vi "Cooling monitor.vi"() -> ()   [LabVIEW 2024]
panel:
  out "Humidity":dbl
  out "Fan steps":dbl
  out "Max Temp":dbl
  out "Min Temp":dbl
  out "Get Arduino Data":bool
  out "Fan Status":bool
  out "Waveform Chart":cluster{"x+y":dbl, dbl, dbl}(graph)
  out "Humidity":dbl(slide) scale=0.0..100.0 scale format="%.0p"
  out "Thermometer":dbl(slide) scale=0.0..100.0
  out "Fan status":string
  out "Humidity":string
  out "Temp":string
  out "Date and time":string
  in  "stop":bool
  out "error out":errorcluster
  out "read buffer":string
  in  "VISA resource name":refnum<visa-resource-name>="COM7"
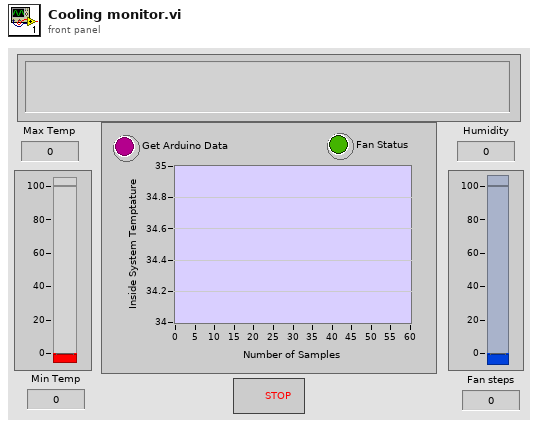
[diagram p1: front panel]
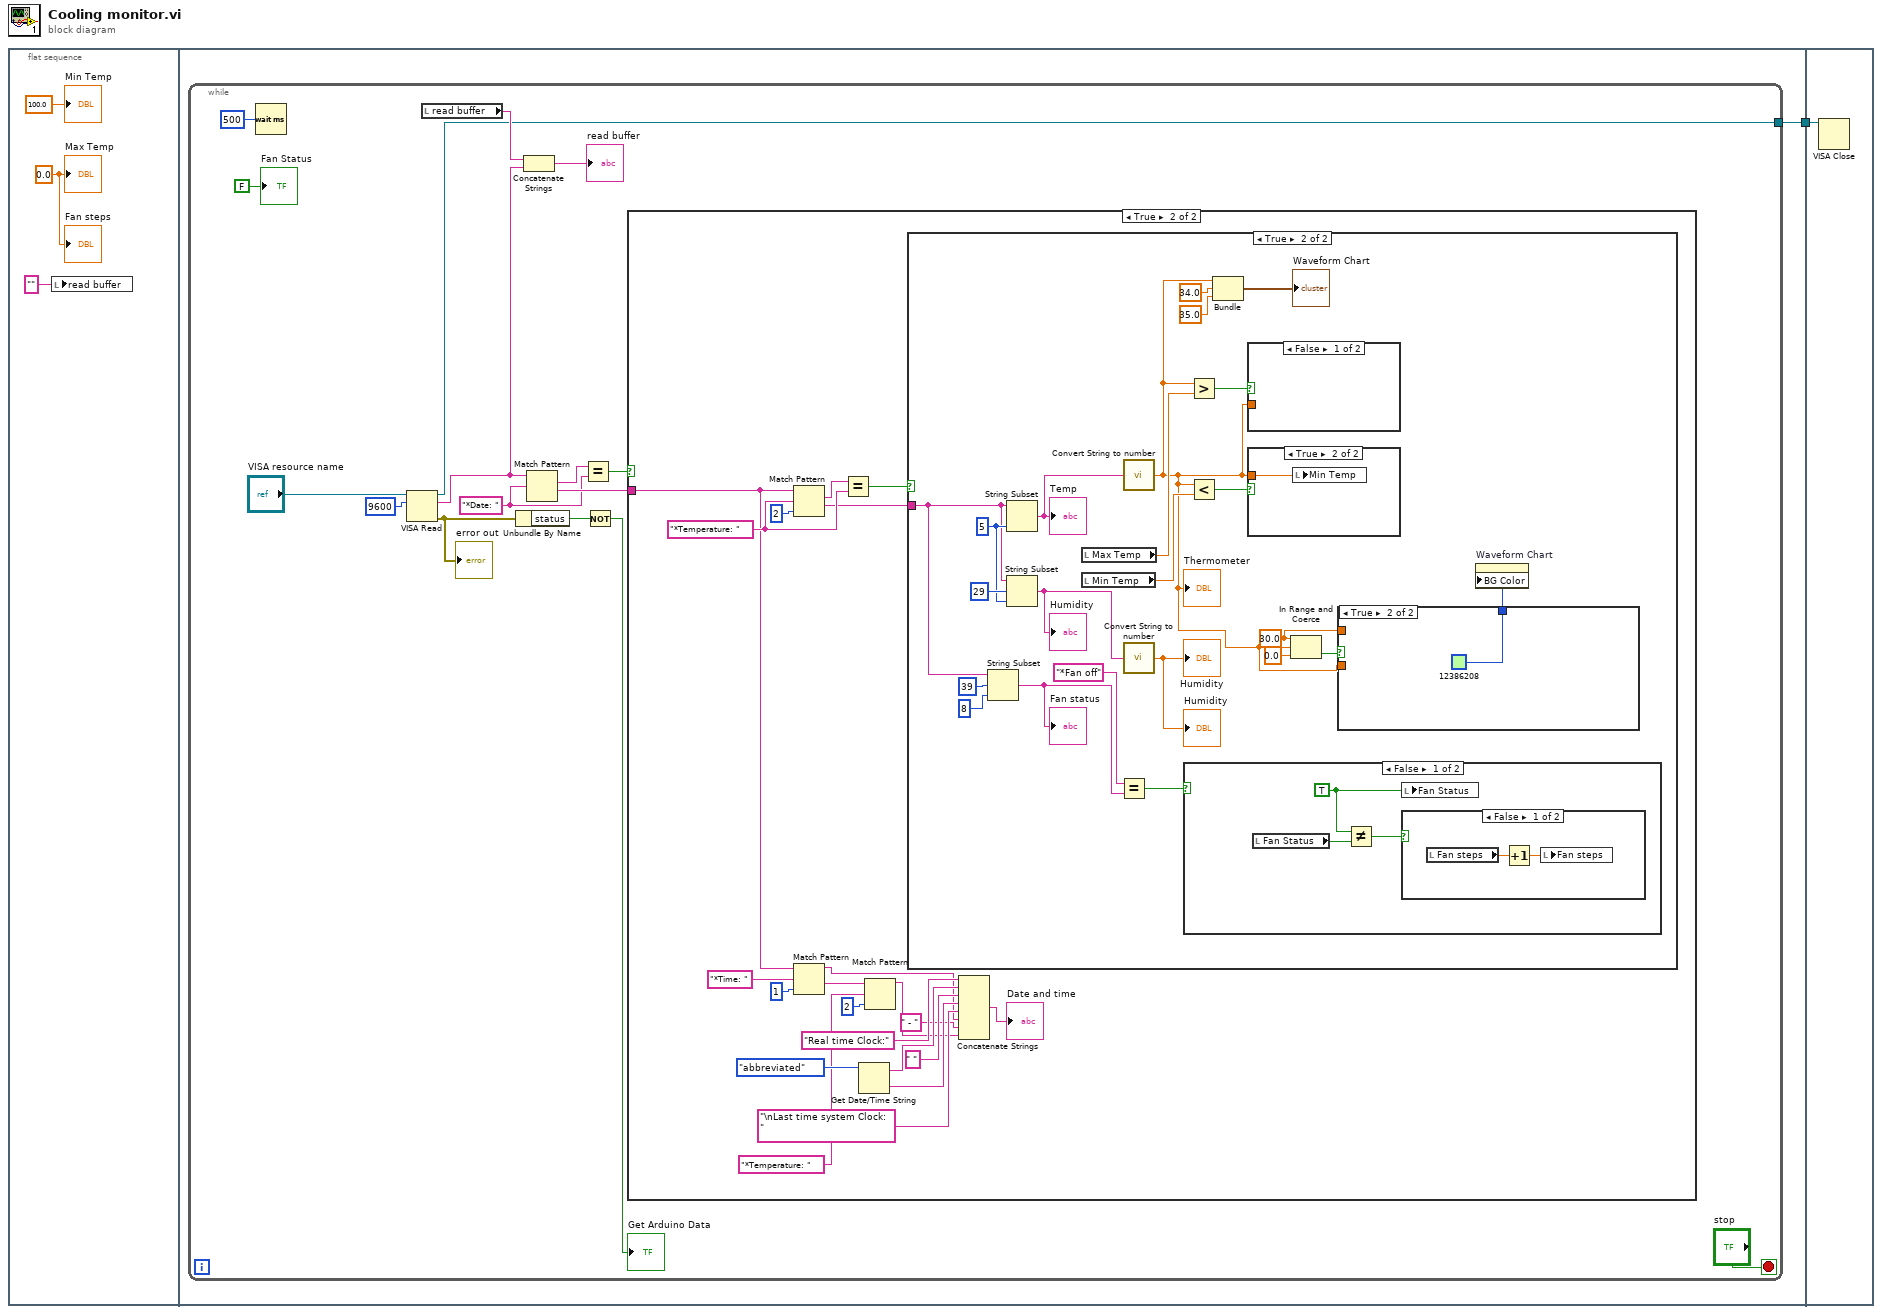
[diagram p0: block diagram]
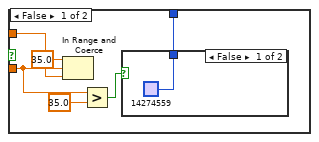
[diagram p4: hidden frame]
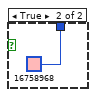
[diagram p5: hidden frame]
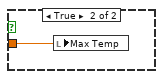
[diagram p7: hidden frame]
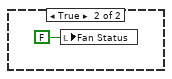
[diagram p9: hidden frame]
diagram:
  n1 = flat-sequence {
    tunnel: [w5] -> w1
    tunnel: w1 -> [w83]
    frame #0 {
      w2 = 0.0 ("Max Temp")
      n2 = local write "read buffer"("" ("read buffer")) -> ()
      "Min Temp" <- 100.0 ("Min Temp")
      "Max Temp" <- w2
      "Fan steps" <- w2
    }
    frame #1 {
      n3 = while {
        tunnel: [w16] -> w5
        stop <- "stop" stop-if-true
        w13 = "*Date: "
        n4 = Wait (ms)(milliseconds to wait=u32 500) -> ()  [unwired: 1 out]
        n5 = VISA Read(VISA resource name="VISA resource name", byte count=u32 9600) -> (VISA resource name out=w16:refnum<visa-resource-name>, read buffer=w15:string, error out=w9:errorcluster)  [unwired: 1 in, 1 out]
        "error out" <- w9
        n6 = local read "read buffer"() -> (w17:string)
        n7 = Unbundle By Name(w9) -> ("status"=w8:bool)
        n8 = Concatenate Strings(w17, w15) -> (→"read buffer":string)
        n9 = Match Pattern(string=w15, regular expression=w13) -> (match substring=w12:string, after substring=w14:string)  [unwired: 1 in, 2 out]
        n10 = Equal?(x=w12, y=w13) -> (x = y?=w11:bool)
        n11 = Not(x=w8) -> (.not. x?=→"Get Arduino Data":bool)
        n12 = case shown="True" w11 {
          tunnel: w14 -> [_ w31]
          frame False {
          }
          frame True {
            w41 = "*Temperature: " ("regular expression")
            n13 = Match Pattern(string=w31, regular expression=w41, offset (0)=2) -> (match substring=w42:string, after substring=w39:string)  [unwired: 2 out]
            n14 = Match Pattern(string=w31, regular expression="*Time: ", offset (0)=1) -> (before substring=w29:string, after substring=w28:string)  [unwired: 2 out]
            n15 = Equal?(x=w42, y=w41) -> (x = y?=w40:bool)
            n16 = Get Date/Time String(date format (0)=enum16{"short", "long", "abbreviated"}."abbreviated") -> (date string=w38:string, time string=w36:string)  [unwired: 2 in]
            n17 = Match Pattern(string=w28, regular expression="*Temperature: ", offset (0)=2) -> (before substring=w25:string)  [unwired: 3 out]
            n18 = case shown="True" w40 {
              tunnel: w39 -> [_ w50]
              frame False {
              }
              frame True {
                w45 = 30.0 ("upper limit")
                w52 = 5 ("length (rest)")
                n19 = String Subset(string=w50, offset (0)=39, length (rest)=8 ("length (rest)")) -> (substring=w51:string)
                "Fan status" <- w51
                n20 = String Subset(string=w50, length (rest)=w52) -> (substring=w55:string)  [unwired: 1 in]
                "Temp" <- w55
                n21 = String Subset(string=w50, offset (0)=29, length (rest)=w52) -> (substring=w54:string)
                "Humidity" <- w54
                n22 = local read "Max Temp"() -> (w62:dbl)
                n23 = local read "Min Temp"() -> (w59:dbl)
                n24 = Equal?(x="*Fan off", y=w51) -> (x = y?=w65:bool)
                n25 = call "Convert String to number.vi"("String"=w55) -> ("x+y"=w44:dbl)
                "Thermometer" <- w44
                n26 = call "Convert String to number.vi"("String"=w54) -> ("x+y"=→"Humidity" →"Humidity":dbl)
                n27 = case shown="False" w65 {
                  frame False {
                    w77 = TRUE ("x")
                    n28 = local read "Fan Status"() -> (w79:bool)
                    n29 = Not Equal?(x=w77, y=w79) -> (x != y?=w78:bool)
                    n30 = local write "Fan Status"(w77) -> ()
                    n31 = case shown="False" w78 {
                      frame False {
                        n32 = local read "Fan steps"() -> (w80:dbl)
                        n33 = Increment(x=w80) -> (x+1=w81:dbl)
                        n34 = local write "Fan steps"(w81) -> ()
                      }
                      frame True {
                      }
                    }
                  }
                  frame True {
                    n35 = local write "Fan Status"(FALSE) -> ()
                  }
                }
                n36 = Greater?(x=w44, y=w62) -> (0:w61:bool)
                n37 = Less?(x=w44, y=w59) -> (x < y?=w60:bool)
                n38 = Bundle("x+y"=w44, 34.0, 35.0) -> (→"Waveform Chart":cluster{"x+y":dbl, dbl, dbl})  [unwired: 1 in]
                n39 = case shown="False" w61 {
                  tunnel: w44 -> [_ w76]
                  frame False {
                  }
                  frame True {
                    n40 = local write "Max Temp"(w76) -> ()
                  }
                }
                n41 = case shown="True" w60 {
                  tunnel: w44 -> [_ w75]
                  frame False {
                  }
                  frame True {
                    n42 = local write "Min Temp"(w75) -> ()
                  }
                }
                n43 = In Range and Coerce(upper limit=w45, x=w44, lower limit=0.0) -> (In Range?=w47:bool)  [unwired: 1 out]
                n44 = case shown="True" w47 {
                  tunnel: w45 -> [w71 _]
                  tunnel: w44 -> [w69 _]
                  tunnel: [w66 u32 12386208 ("Plot Area:Colors:BG Color 2")] -> w43
                  frame False {
                    n45 = In Range and Coerce(upper limit=35.0, x=w69, lower limit=w71) -> ()  [unwired: 2 out]
                    n46 = Greater?(x=w69, y=35.0) -> (0:w67:bool)
                    n47 = case shown="False" w67 {
                      tunnel: [u32 14274559 ("Plot Area:Colors:BG Color 2") u32 16758968 ("Plot Area:Colors:BG Color 2")] -> w66
                      frame False {
                      }
                      frame True {
                      }
                    }
                  }
                  frame True {
                  }
                }
                n48 = property on="Waveform Chart" class="WFChart (strict)"("BG Color"=w43) -> ()  [unwired: 2 in, 2 out]
              }
            }
            n49 = Concatenate Strings("Real time Clock:" ("string"), w38, " " ("string"), w36, "\nLast time system Clock:  " ("string"), w29, " - " ("string"), w25) -> (→"Date and time":string)
          }
        }
        "Fan Status" <- FALSE ("FAN")
      }
    }
    frame #2 {
      n50 = VISA Close(VISA resource name=w83) -> ()  [unwired: 1 in, 1 out]
    }
  }
